vi "LVClass_WavefrontCorrector Assert Equal User Preferences.vi"(0 "WavefrontCorrector in":refnum<class "WavefrontCorrector.lvclass">, 5 "Wavefront Corrector State":T1[](array[typedef]), 7 "Sleep after command apply (ms)":i32, 11 "error in (no error)":errorcluster) -> (4 "WavefrontCorrector out":refnum<class "WavefrontCorrector.lvclass">, 15 "error out":errorcluster)   [LabVIEW 2020, in "WavefrontCorrector.lvclass"]
doc: "Assert requested preferences are equal to current preferences.\n\n--------------------------------------------------------------------------------\n\n<B>correctorIn </B> : WavefrontCorrector object.\n<B>correctorOut </B> : WavefrontCorrector object.\n<B>sleep_after_movement </B> : WavefrontCorrector preferences : Time to stabilization (ms).\n<B>min </B> : WavefrontCorrector preferences : lowest command value.\n<B>max </B> : WavefrontCorrector preferences : highest command value.\n<B>validity </B> : WavefrontCorrector preferences : status.\n<B>fixed_values </B> : WavefrontCorrector preferences : fixed positions.\n<B>ErrorIn </B> : Error\n<B>ErrorOut </B> : Error\n\n--------------------------------------------------------------------------------"
uses:
  WavefrontCorrector.lvclass
  Wavefront Corrector states - ONE.ctl
  WavefrontCorrector.lvclass/WavefrontCorrector.ctl
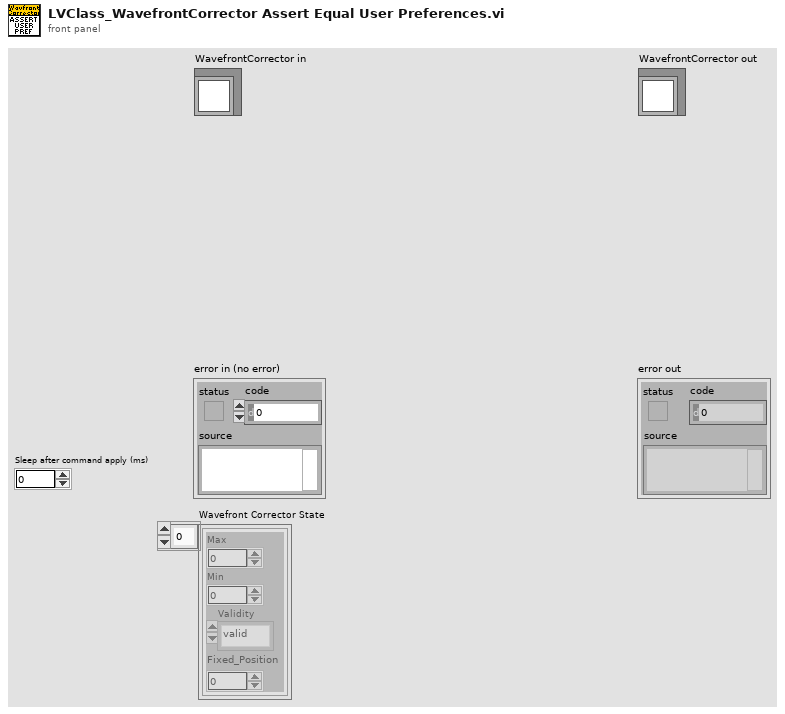
[diagram p1: front panel]
types:
  T1 = typedef "Wavefront Corrector states - ONE.ctl" = cluster{"Max":sgl, "Min":sgl, "Validity":enum16{"valid", "fixed", "invalid"}, "Fixed_Position":sgl}
  T2 = typedef "ClassID.ctl" = i64
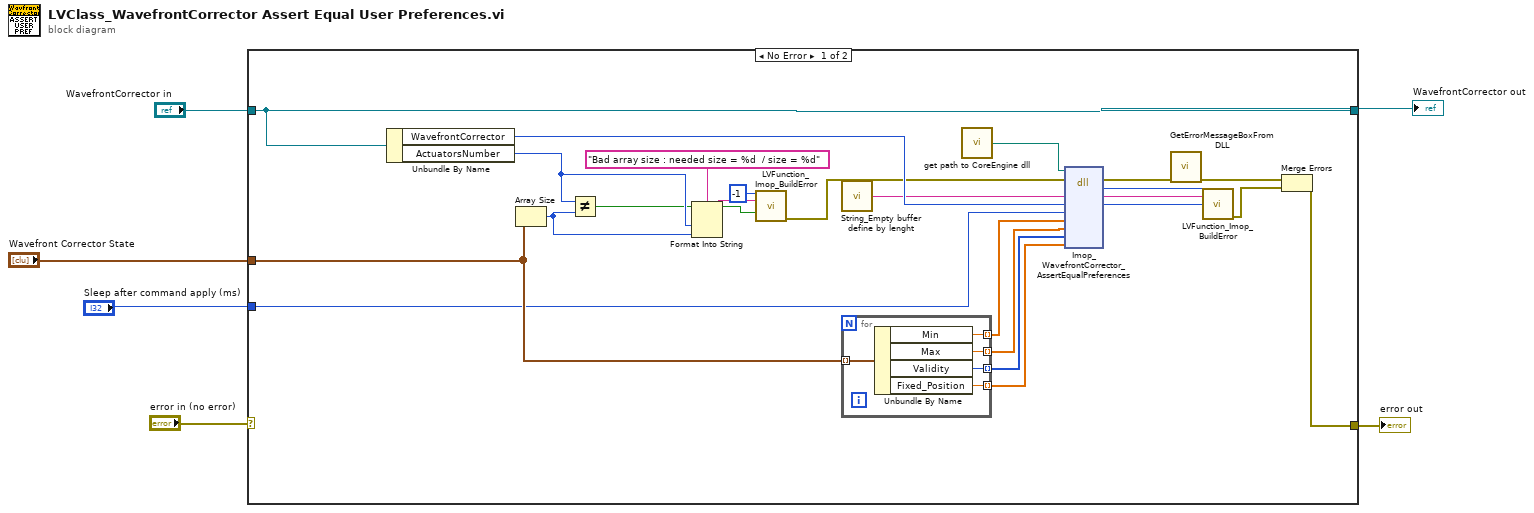
[diagram p0: block diagram]
diagram:
  n1 = case shown="No Error" "error in (no error)" {
    selector: "error in (no error)" -> [_ w37]
    tunnel: [w28 w37] -> w3
    tunnel: [w8 w36] -> w4
    tunnel: "WavefrontCorrector in" -> [w8 w36]
    tunnel: "Wavefront Corrector State" -> [w10 _]
    tunnel: "Sleep after command apply (ms)" -> [w9 _]
    frame No Error {
      n2 = Unbundle By Name(w8) -> ("WavefrontCorrector"=w27:T2, "ActuatorsNumber"=w20:i32)
      n3 = Array Size(array=w10) -> (size(s)=w21:i32)
      n4 = Not Equal?(x=w20, y=w21) -> (x != y?=w15:bool)
      n5 = Format Into String(format string="Bad array size : needed size = %d  / size = %d" ("String to Prepend to source (\"\")"), w20, w21) -> (resulting string=w22:string)  [unwired: 2 in, 1 out]
      n6 = call "LVFunction_Imop_BuildError.vi"("code"=-1, "String to Prepend to source (\"\")"=w22, "Activate error? (true)"=w15) -> ("error out"=w13:errorcluster)  [unwired: 12 in]
      n7 = call "String_Empty buffer define by lenght.vi"() -> ("Empty buffer"=w18:string)  [unwired: 1 in]
      n8 = for {
        tunnel: w10 -> [w35] mode=indexing
        tunnel: [w34] -> w12 mode=indexing
        tunnel: [w33] -> w11 mode=indexing
        tunnel: [w32] -> w17 mode=indexing
        tunnel: [w31] -> w16 mode=indexing
        n9 = Unbundle By Name(w35) -> ("Min"=w34:sgl, "Max"=w33:sgl, "Validity"=w32:enum16{"valid", "fixed", "invalid"}, "Fixed_Position"=w31:sgl)
      }
      n10 = call "get path to CoreEngine dll.vi"() -> ("path to wavekit library"=w19:path)  [unwired: 14 in, 1 out]
      n11 = dll-call lib="D:/soft/HASO_v3/SVN_trunk/ImOpCoreEngine4_LV2011/DLLs/c_interface_vc100.dll" fn="Imop_WavefrontCorrector_AssertEqualPreferences"(path in=w19, error in=w13, "message"=w18, "WavefrontCorrection"=w27, "sleep_after_movement"=w9, "min"=w12, "max"=w11, "validity"=w17, "fixed_value"=w16) -> (error out=w26:errorcluster, "return type"=w25:i32, "message"=w24:string, "WavefrontCorrection"=w7:i64)  [unwired: 6 in, 1 out]
      n12 = call "GetErrorMessageBoxFromDLL.vi"("error IN"=w26) -> ("error OUT"=w30:errorcluster)  [unwired: 10 in]
      n13 = call "LVFunction_Imop_BuildError.vi"("code"=w25, "String to Prepend to source (\"\")"=w24, "Adresse"=w7) -> ("error out"=w29:errorcluster)  [unwired: 12 in]
      n14 = Merge Errors(w30, w29) -> (w28:errorcluster)
    }
    frame Error {
    }
  }
  "error out" <- w3
  "WavefrontCorrector out" <- w4
